vi "Test Convert.vi"(11 "Error in":errorcluster) -> (15 "Error out":errorcluster)   [LabVIEW 2020, in "CelsiusToFarenheitTests.lvlib"]
doc: "This VI is to validate Celsius to farenheit"
uses:
  CelsiusToFarenheitTests.lvlib
  <vilib>/SLL Drona/APIs/Stimulus/ControlValue/ValueSignalByPathString.vi
  <vilib>/SLL Drona/APIs/Assert/AssertControlValue/AlmostEqual.vi
  <vilib>/SLL Drona/APIs/Stimulus/VI/CloseVI.vi
  <vilib>/Utility/error.llb/Error Cluster From Error Code.vi
  <vilib>/ErrorRing/Error Ring.xnode
  <vilib>/SLL Drona/Drona.lvlib
  <vilib>/addons/_JKI Toolkits/Caraya/classes/Test/Test.lvclass
  <vilib>/Wiresmith Technology/G CLI/CLI Class/CLI.lvclass
  <vilib>/SLL Drona/APIs/Stimulus/VI/VI.lvlib
  <vilib>/SLL Drona/APIs/Assert/AssertControlValue/AssertControlValue.lvlib
  <vilib>/SLL Drona/APIs/Stimulus/ControlValue/ControlValue.lvlib
panel:
  # "CELSIUS TO FAHRENHEIT TEST"
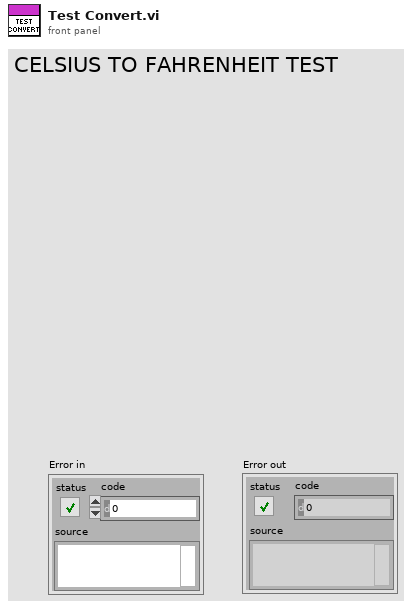
[diagram p1: front panel]
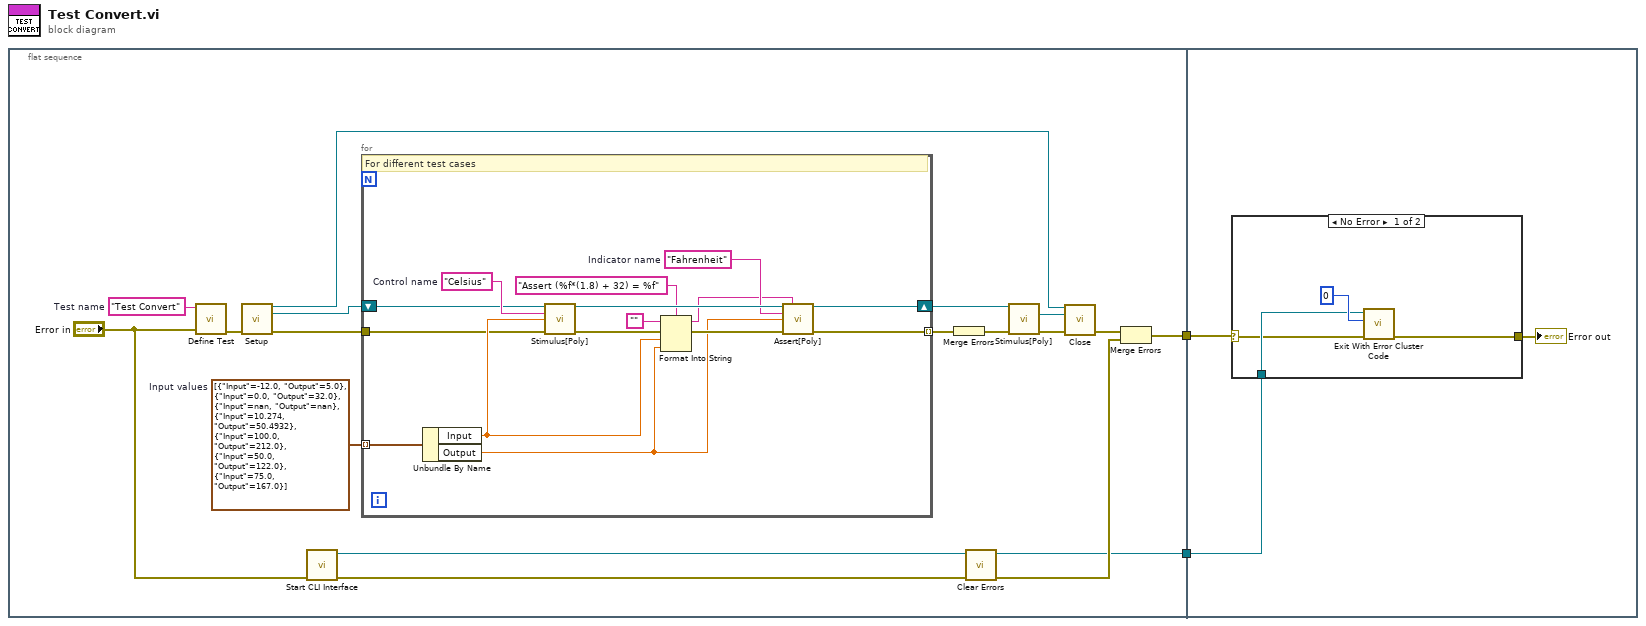
[diagram p0: block diagram]
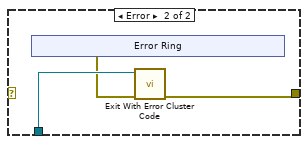
[diagram p2: hidden frame]
diagram:
  n1 = flat-sequence {
    tunnel: [w4] -> w2
    tunnel: [w5] -> w1
    tunnel: w2 -> [w35]
    tunnel: w1 -> [w37]
    frame #0 {
      w9 = "Test Convert"  # Test name
      w19 = cluster{"Input":dbl, "Output":dbl}[] [{"Input"=-12.0, "Output"=5.0}, {"Input"=0.0, "Output"=32.0}, {"Input"=nan, "Output"=nan}, {"Input"=10.274, "Output"=50.4932}, {"Input"=100.0, "Output"=212.0}, {"Input"=50.0, "Output"=122.0}, {"Input"=75.0, "Output"=167.0}]  # Input values
      n2 = call <vilib>:"Define Test.vi"("error in (no error)"="Error in", "Label (VI Title)"=w9) -> ("error out"=w10:errorcluster)  [unwired: 9 in]
      n3 = call <vilib>:"Setup.vi"("error in"=w10) -> ("Application Ref"=w17:refnum<vi>, "VI Reference Out"=w18:refnum<vi>, "error out"=w12:errorcluster)  [unwired: 12 in]
      n4 = call <vilib>:"Start CLI Interface.vi"("error in (no error)"="Error in") -> ("error out"=w3:errorcluster, "CLI out"=w4:refnum<class "CLI.lvclass">)  [unwired: 7 in, 2 out]
      n5 = for {
        tunnel: w19 -> [w34] mode=indexing
        shift-right: [w24] -> w16
        shift-left: w18 -> [w32]
        tunnel: w12 -> [w21]
        tunnel: [w20] -> w14 mode=indexing
        w25 = "Fahrenheit"  # Indicator name
        w33 = "Celsius"  # Control name
        # "For different test cases"
        n6 = Unbundle By Name(w34) -> ("Input"=w22:dbl, "Output"=w26:dbl)
        n7 = call-poly <vilib>:"Stimulus[Poly].vi"("VI Reference In"=w32, "Control Path"=w33, "Value (Signaling)"=w22, "error in"=w21) -> ("VI Reference Out"=w28:refnum<vi>, "error out"=w30:errorcluster)  [unwired: 10 in]
        n8 = Format Into String(format string="Assert (%f*(1.8) + 32) = %f", initial string="", error in=w30, w22, w26) -> (resulting string=w23:string, error out=w29:errorcluster)
        n9 = call-poly <vilib>:"Assert[Poly].vi"("VI Reference In"=w28, "Test Label"=w23, "Control Path"=w25, "Control Value"=w26, "Error In"=w29) -> ("VI Reference Out"=w24:refnum<vi>, "Error Out"=w20:errorcluster)  [unwired: 9 in]
      }
      n10 = Merge Errors(w14) -> (w11:errorcluster)
      n11 = call <vilib>:"Clear Errors.vi"("error in (no error)"=w3) -> ("error out"=w6:errorcluster)  [unwired: 5 in, 1 out]
      n12 = call-poly <vilib>:"Stimulus[Poly].vi"("VI Reference In"=w16, "error in"=w11) -> ("VI Reference Out"=w15:refnum<vi>, "error out"=w13:errorcluster)  [unwired: 12 in]
      n13 = call <vilib>:"Close.vi"("Application Ref"=w17, "VI Reference"=w15, "error in"=w13) -> ("error out"=w7:errorcluster)  [unwired: 12 in]
      n14 = Merge Errors(w7, w6) -> (w5:errorcluster)
    }
    frame #1 {
      n15 = case shown="No Error" w37 {
        selector: w37 -> [w38 _]
        tunnel: [w40 w44] -> w36
        tunnel: w35 -> [w39 w43]
        frame No Error {
          n16 = call <vilib>:"Exit With Error Cluster Code.vi"("error in (no error)"=w38, "No Error Code (0)"=0, "CLI in"=w39) -> ("error out"=w40:errorcluster)  [unwired: 8 in]
        }
        frame Error {
          n17 = xnode "Error Ring"() -> ("error out"=w42:errorcluster)
          n18 = call <vilib>:"Exit With Error Cluster Code.vi"("error in (no error)"=w42, "CLI in"=w43) -> ("error out"=w44:errorcluster)  [unwired: 9 in]
        }
      }
      "Error out" <- w36
    }
  }
